vi "Gen_StartSample.vi"(8 "错误输入":errorcluster caption="错误输入（无错误）", 10 "Cards":T1[](array[typedef]), 11 "QXDAQ reference":refnum<k24>) -> (0 "错误输出":errorcluster)   [LabVIEW 2016]
uses:
  DAQ-Config/Controls/PSCHN_Channel Para.ctl
  DAQ-Config/Controls/PSCHN_Card Para.ctl
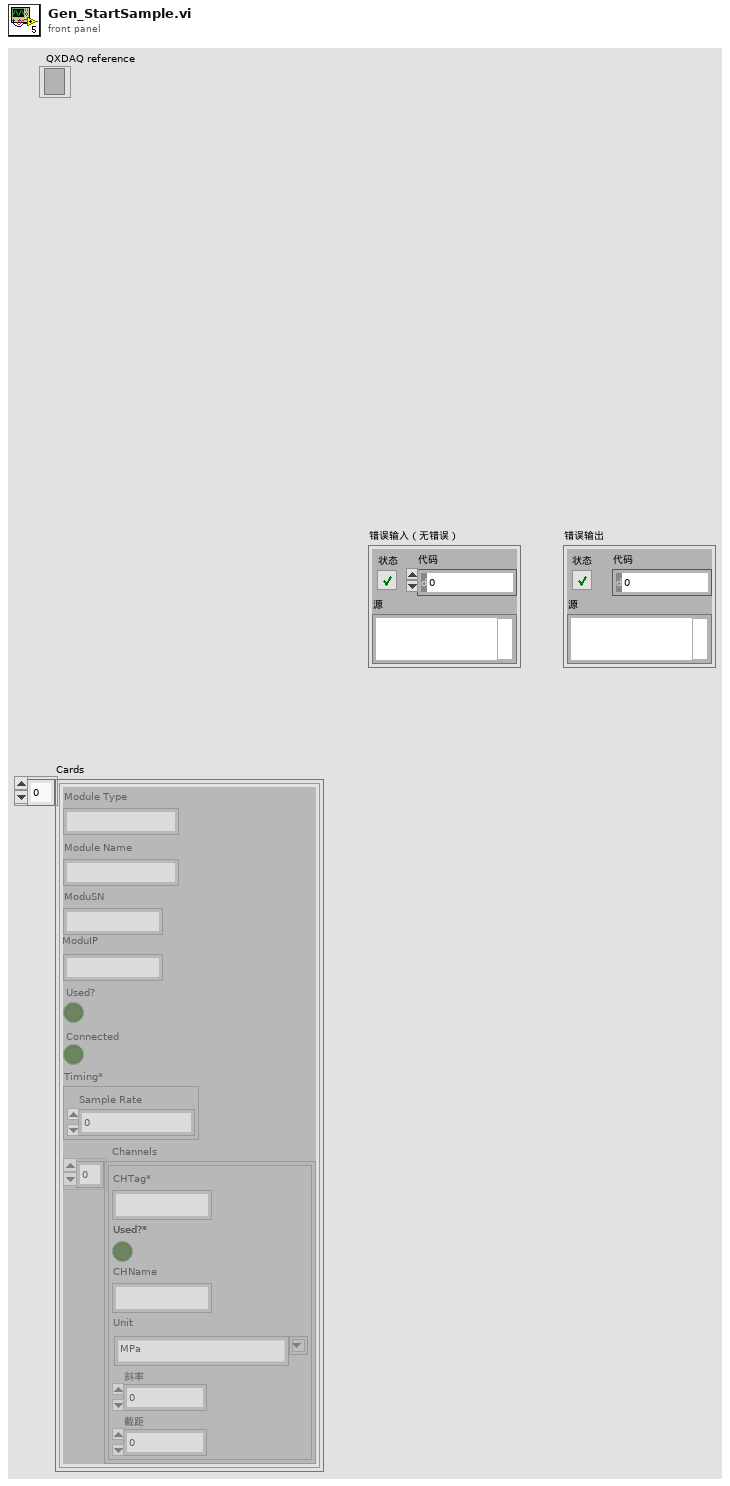
[diagram p1: front panel]
types:
  T1 = typedef "PSCHN_Card Para.ctl" = cluster{"Module Type":string, "Module Name":string, "ModuSN":string, "ModuIP":string, "Used?":bool, "Connected":bool, "Timing*":cluster{"Sample Rate":dbl}, "Channels":T2[]}
  T2 = typedef "PSCHN_Channel Para.ctl" = cluster{"CHTag*":string, "Used?*":bool, "CHName":string, "Unit":string, "斜率":dbl, "截距":dbl}
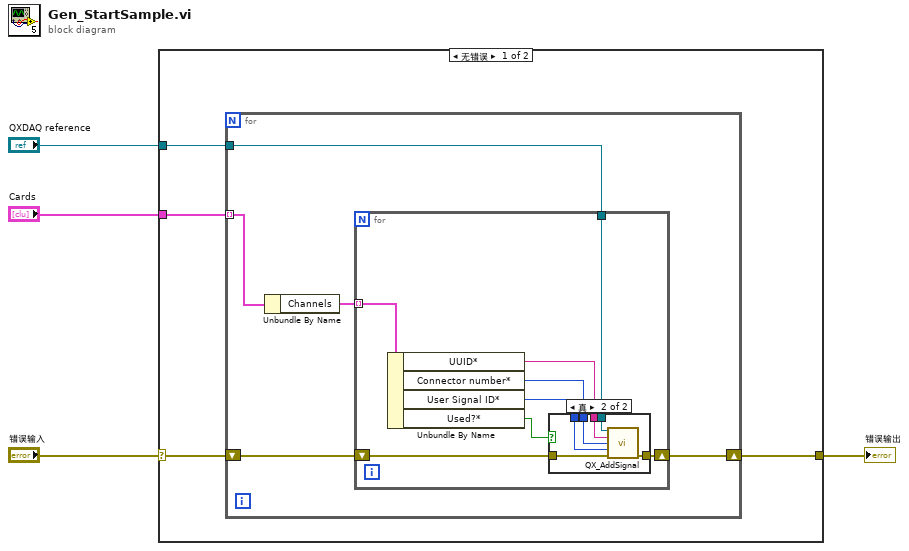
[diagram p0: block diagram]
diagram:
  n1 = case shown="无错误" "错误输入" {
    selector: "错误输入" -> [w7 w29]
    tunnel: [w6 w29] -> w3
    tunnel: "Cards" -> [w8 _]
    tunnel: "QXDAQ reference" -> [w5 _]
    frame No Error {
      n2 = for {
        tunnel: w8 -> [w13] mode=indexing
        shift-right: [w11] -> w6
        shift-left: w7 -> [w12]
        tunnel: w5 -> [w10]
        n3 = Unbundle By Name(w13) -> ("Channels"=w9:T2[])
        n4 = for {
          shift-right: [w17] -> w11
          shift-left: w12 -> [w18]
          tunnel: w10 -> [w16]
          tunnel: w9 -> [w15] mode=indexing
          n5 = Unbundle By Name(w15) -> ("UUID*"=w21:string, "Connector number*"=w20:i32, "User Signal ID*"=w19:i32, "Used?*"=w14:bool)
          n6 = case shown="真" w14 {
            tunnel: w21 -> [_ w28]
            tunnel: w20 -> [_ w27]
            tunnel: w19 -> [_ w26]
            tunnel: w18 -> [w22 w25]
            tunnel: [w22 w24] -> w17
            tunnel: w16 -> [_ w23]
            frame False {
            }
            frame True {
              n7 = call <userlib>:"QX_AddSignal.vi"("QXDAQ reference"=w23, "UUID"=w28, "Connector number"=w27, "UserSignalID"=w26, "error in"=w25) -> ("error out"=w24:errorcluster)  [unwired: 9 in, 1 out]
            }
          }
        }
      }
    }
    frame Error {
    }
  }
  "错误输出" <- w3
